vi "Adjustable.vi"() -> ()   [LabVIEW 2015]
uses:
  <vilib>/DAQmx/write.llb/DAQmx Write (Analog DBL 1Chan 1Samp).vi
  <vilib>/DAQmx/miscellaneous.llb/DAQmx Fill In Error Info.vi
panel:
  out "error of A1":errorcluster
  out "error of A0":errorcluster
  in  "IamA0 GREEN":refnum<k21>="IamA1"
  in  "IamA1 RED":refnum<k21>="IamA1"
  in  "Stop Button":bool
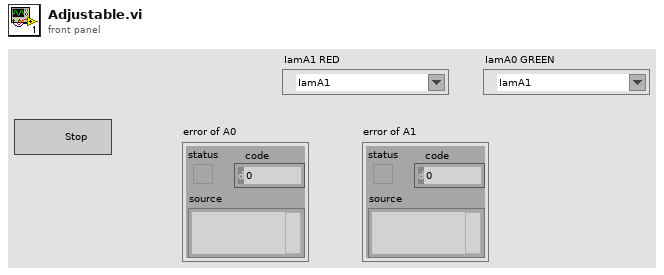
[diagram p1: front panel]
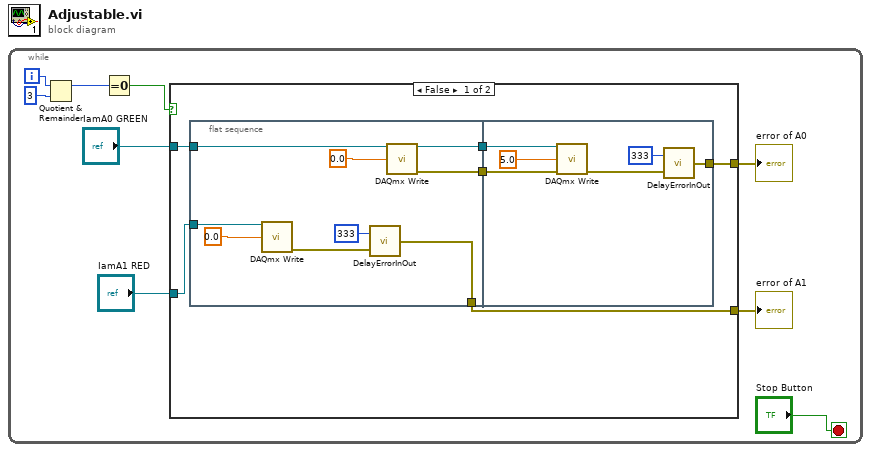
[diagram p0: block diagram]
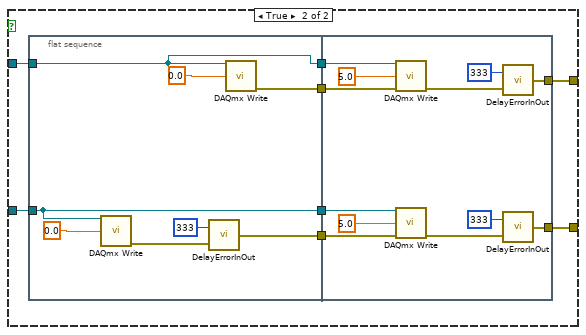
[diagram p2: hidden frame]
diagram:
  n1 = while {
    i -> [w8]
    stop <- "Stop Button" stop-if-true
    n2 = Quotient & Remainder(x=w8, y=3) -> (x-y*floor(x/y)=w6:i32)  [unwired: 1 out]
    n3 = Equal To 0?(x=w6) -> (x = 0?=w5:bool)
    n4 = case shown="False" w5 {
      tunnel: "IamA0 GREEN" -> [w13 w37]
      tunnel: [w10 w36] -> w3
      tunnel: "IamA1 RED" -> [w14 w35]
      tunnel: [w11 w32] -> w1
      frame False {
        n5 = flat-sequence {
          tunnel: [w20] -> w15
          tunnel: w14 -> [w19]
          tunnel: w13 -> [w18]
          tunnel: [w17] -> w12
          tunnel: [w16] -> w11
          tunnel: w15 -> [w27]
          tunnel: w12 -> [w26]
          tunnel: [w25] -> w10
          frame #0 {
            n6 = call-poly <vilib>:"DAQmx Write.vi"("task/channels in"=w19, "data"=0.0 ("Voltage (red)")) -> ("error out"=w21:errorcluster)  [unwired: 11 in, 2 out]
            n7 = call "DelayErrorInOut.vi"("error in"=w21, "milliseconds to wait"=u32 333) -> ("error out"=w16:errorcluster)
            n8 = call-poly <vilib>:"DAQmx Write.vi"("task/channels in"=w18, "data"=0.0 ("Voltage (red)")) -> ("task out"=w17:refnum<k21>, "error out"=w20:errorcluster)  [unwired: 11 in, 1 out]
          }
          frame #1 {
            n9 = call-poly <vilib>:"DAQmx Write.vi"("task/channels in"=w26, "data"=5.0 ("Voltage (red)"), "error in"=w27) -> ("error out"=w28:errorcluster)  [unwired: 10 in, 2 out]
            n10 = call "DelayErrorInOut.vi"("error in"=w28, "milliseconds to wait"=u32 333) -> ("error out"=w25:errorcluster)
          }
        }
      }
      frame True {
        n11 = flat-sequence {
          tunnel: [w42] -> w38
          tunnel: w37 -> [w39]
          tunnel: w35 -> [w40]
          tunnel: [w41] -> w34
          tunnel: [w40] -> w33
          tunnel: [w39] -> w31
          tunnel: w38 -> [w55]
          tunnel: [w54] -> w36
          tunnel: w34 -> [w50]
          tunnel: w33 -> [w49]
          tunnel: [w48] -> w32
          tunnel: w31 -> [w47]
          frame #0 {
            n12 = call-poly <vilib>:"DAQmx Write.vi"("task/channels in"=w40, "data"=0.0 ("Voltage (red)")) -> ("error out"=w43:errorcluster)  [unwired: 11 in, 2 out]
            n13 = call "DelayErrorInOut.vi"("error in"=w43, "milliseconds to wait"=u32 333) -> ("error out"=w41:errorcluster)
            n14 = call-poly <vilib>:"DAQmx Write.vi"("task/channels in"=w39, "data"=0.0 ("Voltage (red)")) -> ("error out"=w42:errorcluster)  [unwired: 11 in, 2 out]
          }
          frame #1 {
            n15 = call-poly <vilib>:"DAQmx Write.vi"("task/channels in"=w47, "data"=5.0 ("Voltage (red)"), "error in"=w55) -> ("error out"=w56:errorcluster)  [unwired: 10 in, 2 out]
            n16 = call-poly <vilib>:"DAQmx Write.vi"("task/channels in"=w49, "data"=5.0 ("Voltage (red)"), "error in"=w50) -> ("error out"=w51:errorcluster)  [unwired: 10 in, 2 out]
            n17 = call "DelayErrorInOut.vi"("error in"=w56, "milliseconds to wait"=u32 333) -> ("error out"=w54:errorcluster)
            n18 = call "DelayErrorInOut.vi"("error in"=w51, "milliseconds to wait"=u32 333) -> ("error out"=w48:errorcluster)
          }
        }
      }
    }
    "error of A0" <- w3
    "error of A1" <- w1
  }
